vi "Master Setup Read Write Update Command.vi"(8 "error in (no error)":errorcluster, 9 "Read (F)/Write (T)":bool, 10 "Pattern Label":T1 items=["Channel Setup (0)", "PID Setup (1)", "Filter Setup (2)", "~Reserved Old CAN Msgs (3)", "~Reserved Old CAN1 (4)", "~Reserved Old CAN2 (5)", "Digital Inputs Setup (6)", "Digital Outputs Setup (7)", "Logging 1 Setup (8)", "Logging 2 Setup (9)", "Logging 3 Setup (10)", "Setpoint Setup (11)", "Test Series Setup (12)", "Graph Setup (13)", "System Configure (14)", "Header (15)", "Profile Manager (16)", "Post-Mortem Logging (17)", "High-Speed Data (18)", "Statistic Channel Setup (19)", "Ramp Channel Setup (20)", "ETAS INCA Channel Setup (21)", "ETC ECCS Transducer Setup (22)", "ETC ECCS Test Setup (23)", "AVL AK Smoke Meter Setup (24)", "Triggers Setup (25)", "Alarm Limits Setup (26)", "YKWT1 Measurement (27)", "YKWT1 Instrument (28)", "Auto File Settings (29)", "Playback File Setting (30)", "UUT Constants (31)", "UPS Setup (32)", "Differential Channel Setup (33)", "Integral Channel Setup (34)", "Signal Channel Setup (35)", "Calibration Setup (36)", "BNC Setup (37)", "ASAP3 Setup (38)", "Chassis Force Calculations (39)", "Chassis Teststand Losses (40)", "Chassis Vehicle Losses (41)", "Formula Channels (42)", "ASAP3 Map Coords Setup (43)", "Digital Controls Setup (44)", "Push Buttons Setup (45)", "Sliders Setup (46)", "~Reserved~ (47)", "Email Setup (48)", "Timer Setup (49)", "Unit Conversion Setup (50)", "Visible Channels (51)", "Main Display Setup (52)", "Message Display Setup (53)", "Input Display Setup (54)", "Unico Parameter Downloads (55)", "Flow Meter Setup (56)", "Channel Zero Offset (57)", "YKWT2 Measurement (58)", "YKWT2 Instrument (59)", "~Reserved Old CAN3 (60)", "CAS Setup (61)", "Accumulation Channel Setup (62)", "Valvetrain Dynamics Setup (63)", "CCP Setup (64)", "System Log Setup (65)", "Throttle Controller (66)", "RE Shifter (67)", "Main Display (68)", "~Reserved~ (69)", "FlexRay (70)", "YKWT3 Measurement (71)", "YKWT3 Instrument (72)", "CAN XNET API (73)"], 11 "Update Command (in)":bool) -> (0 "error out":errorcluster, 3 "Update Command (out)":bool)   [LabVIEW 2017]
uses:
  Master Setup Pattern Enum.ctl
panel:
  in  "Setup File (System Configure)":path=path "C:/Revolutionary Engineering/REPS/Setup Files/Default/GM Trans Cell 2/SystemConfigure GM cell 2.cfs"
  in  "Setup File (Setpoint)":path=path "C:/Revolutionary Engineering/REPS/Setup Files/Default/RE Cell 3-1/re cell 3 setpoints.spt"
  in  "Setup File (CAN 0)":path
  in  "Setup File (CAN 1)":path
  in  "Setup File (Can Message)":path
  in  "Setup File (Playback)":path
  in  "Setup File (UUT Constants)":path
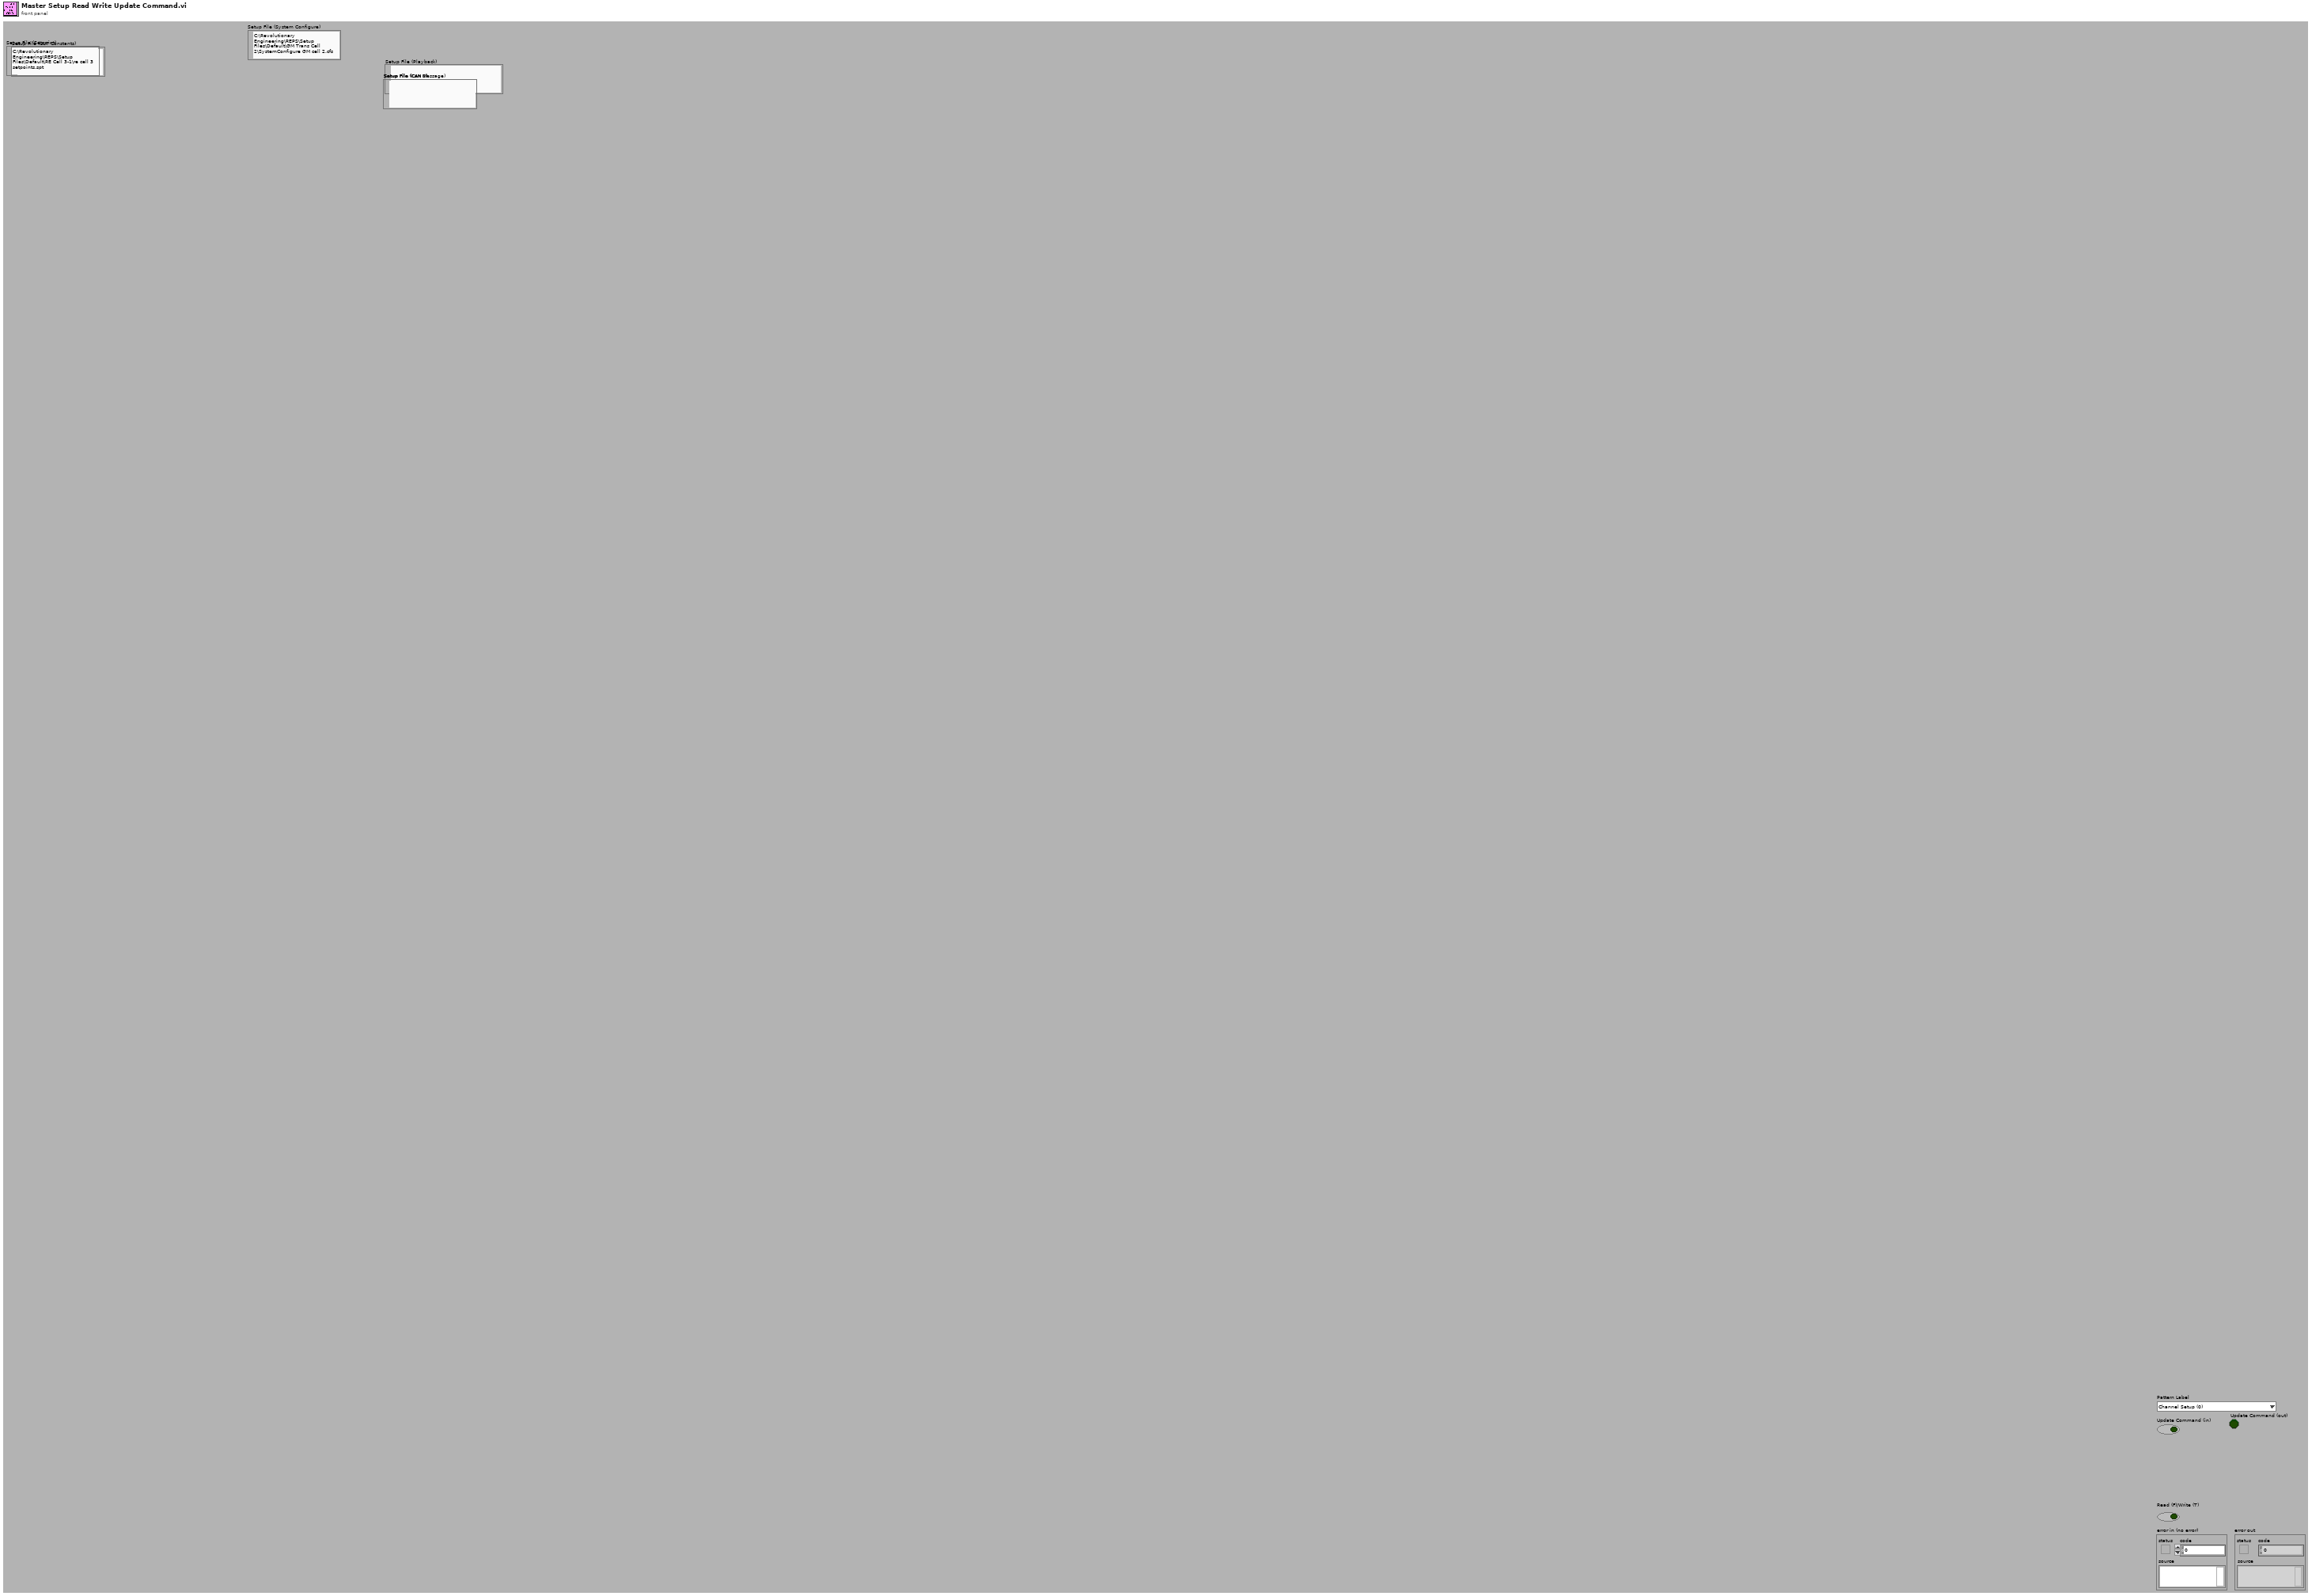
[diagram p1: front panel]
types:
  T1 = typedef "Master Setup Pattern Enum.ctl" = i32
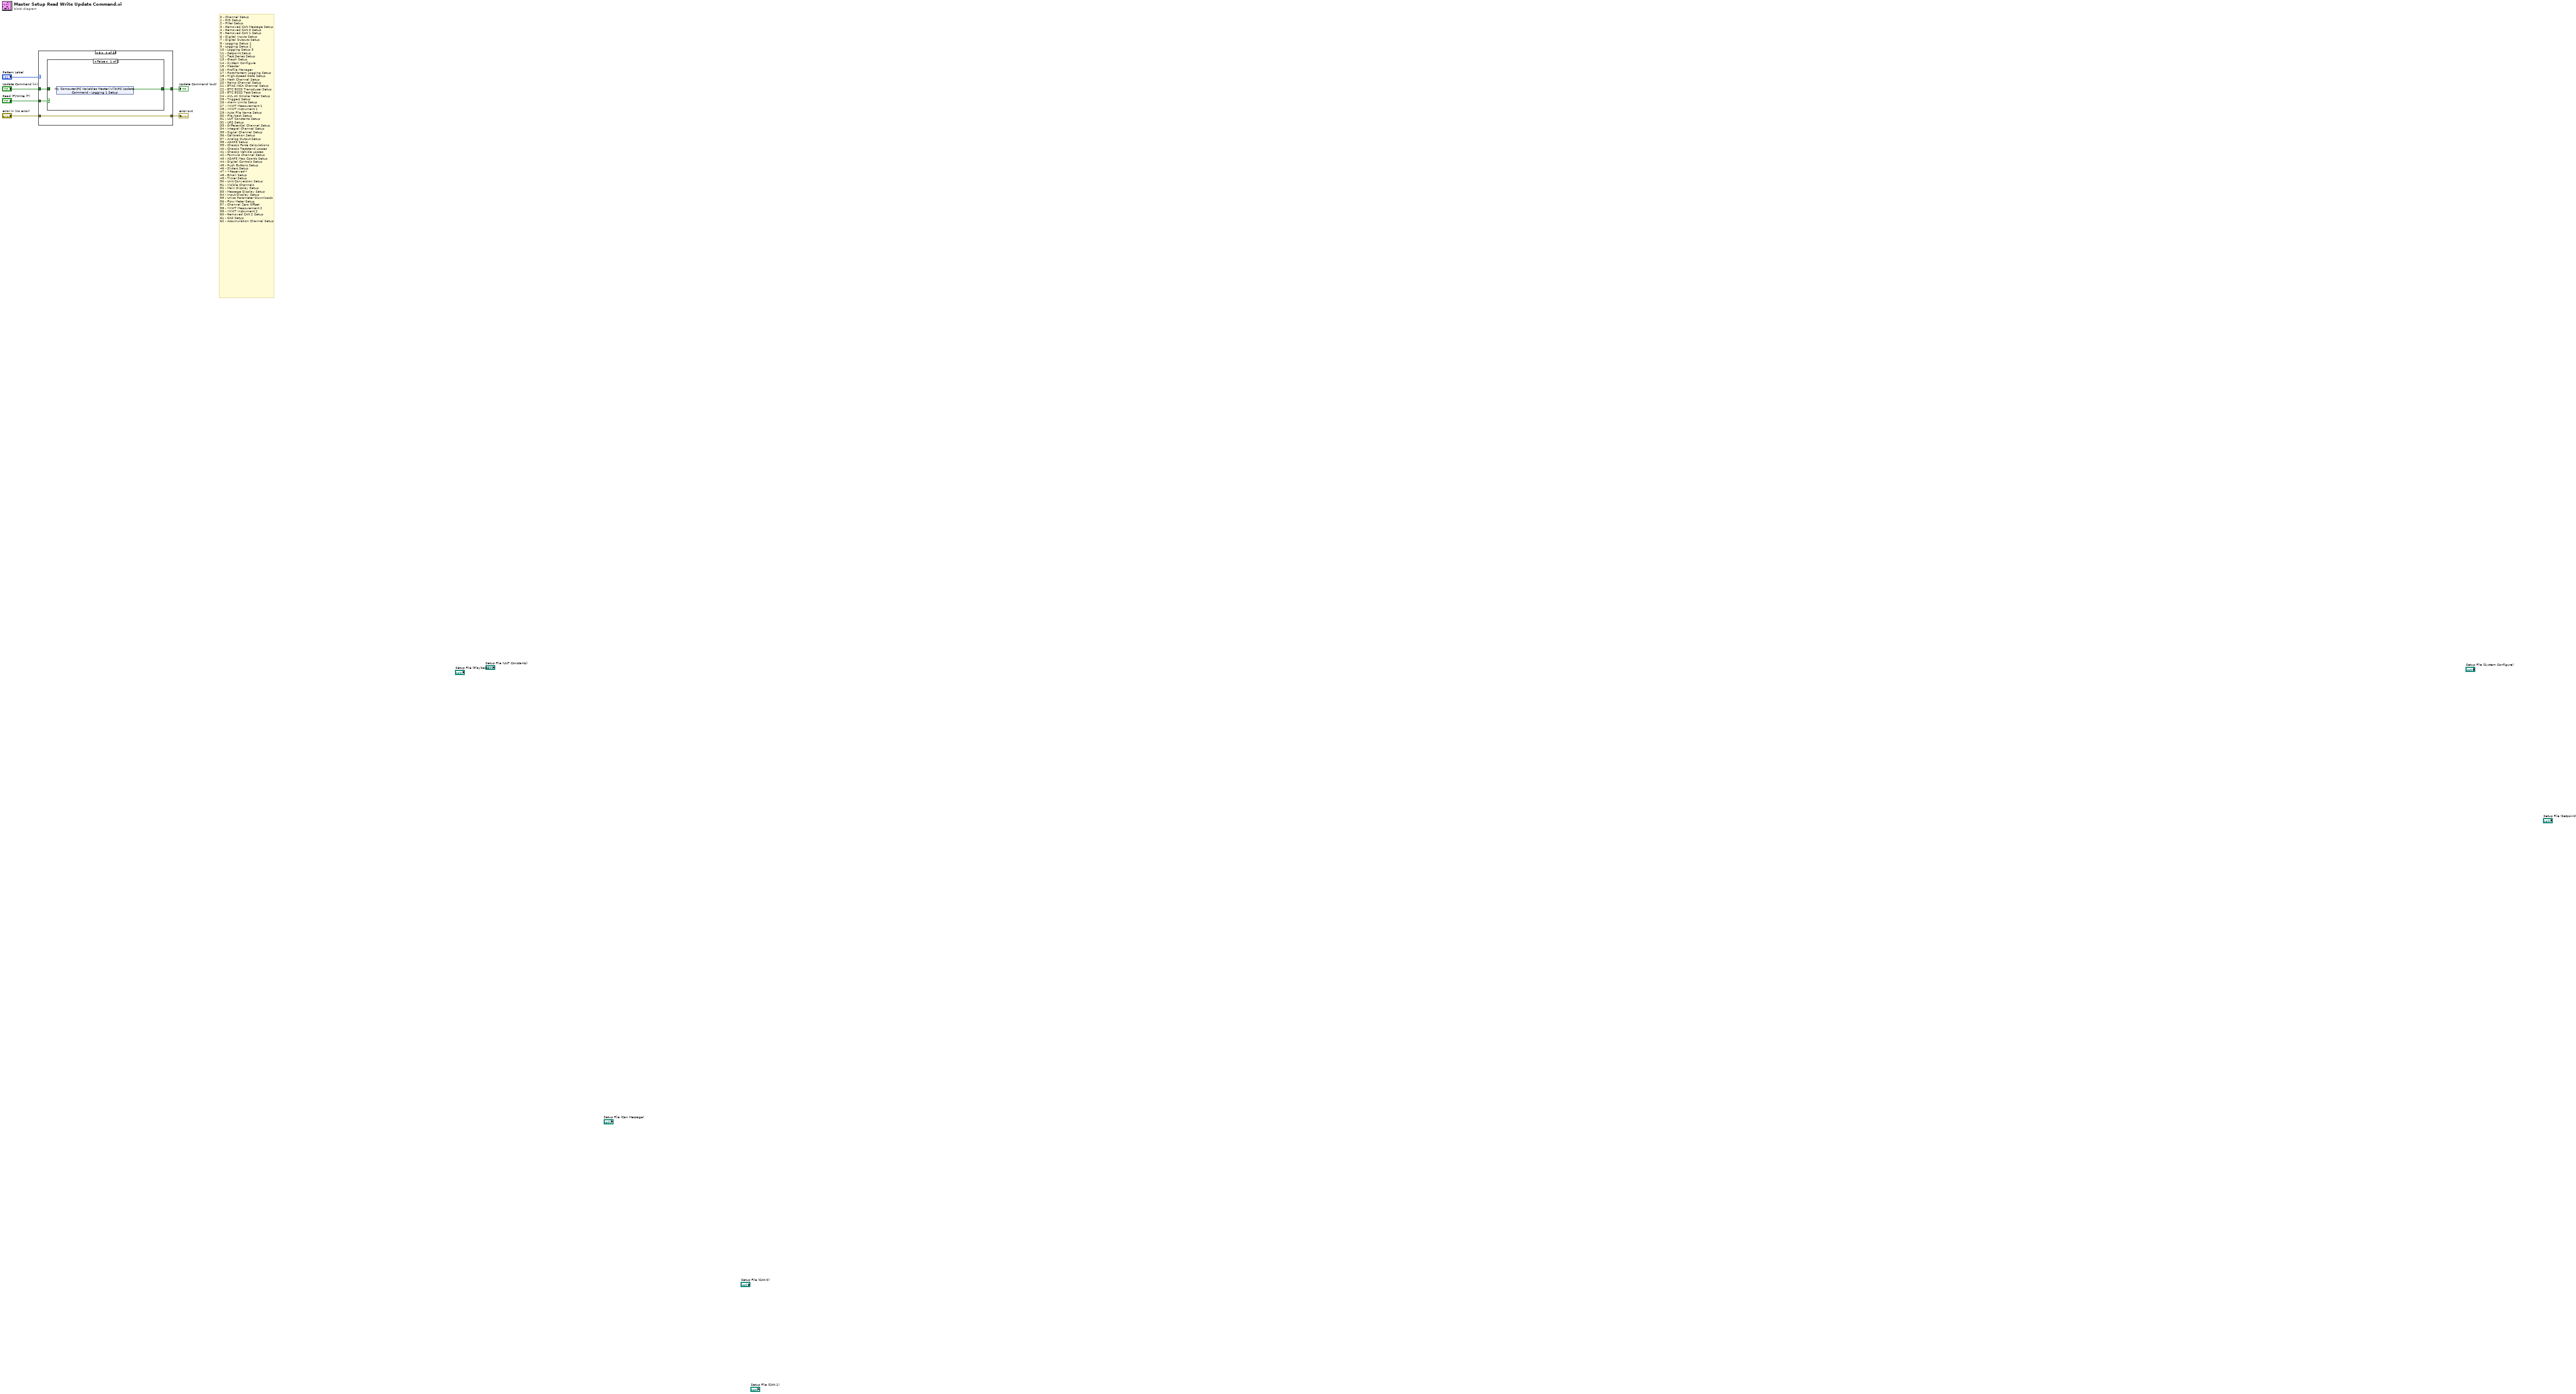
[diagram p0: block diagram]
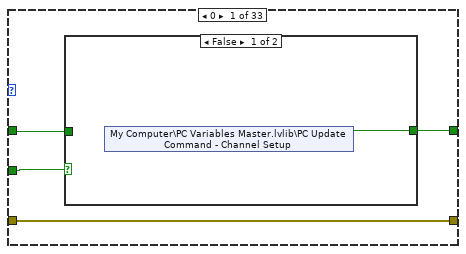
[diagram p2: hidden frame]
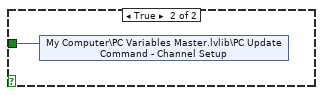
[diagram p3: hidden frame]
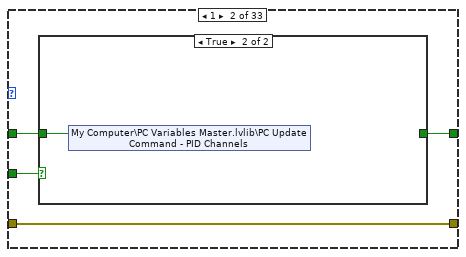
[diagram p4: hidden frame]
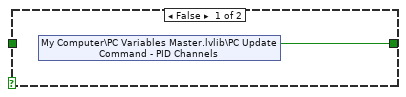
[diagram p5: hidden frame]
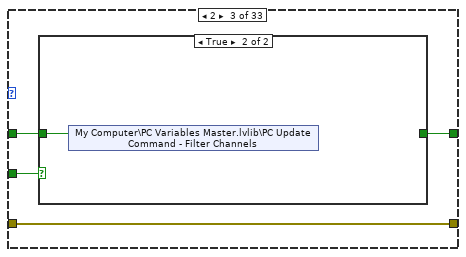
[diagram p6: hidden frame]
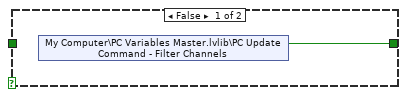
[diagram p7: hidden frame]
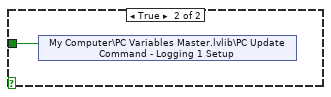
[diagram p8: hidden frame]
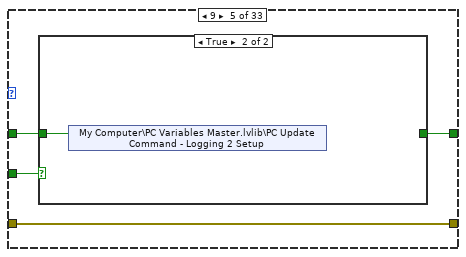
[diagram p9: hidden frame]
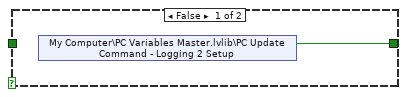
[diagram p10: hidden frame]
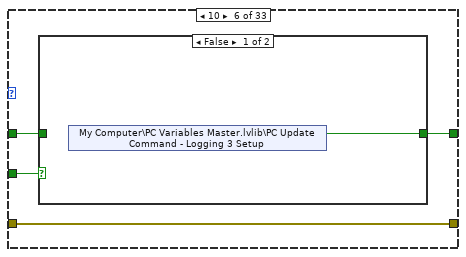
[diagram p11: hidden frame]
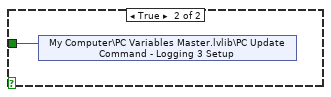
[diagram p12: hidden frame]
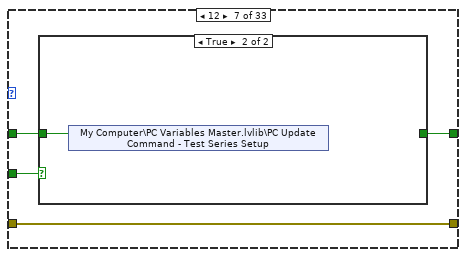
[diagram p13: hidden frame]
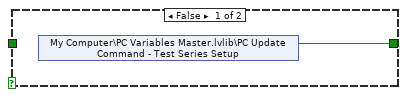
[diagram p14: hidden frame]
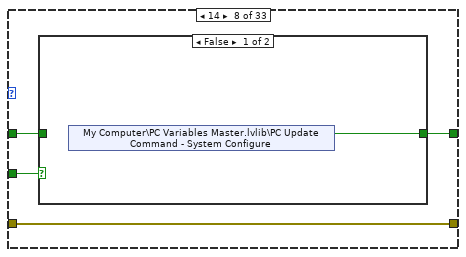
[diagram p15: hidden frame]
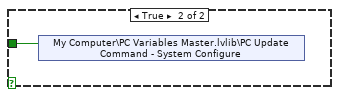
[diagram p16: hidden frame]
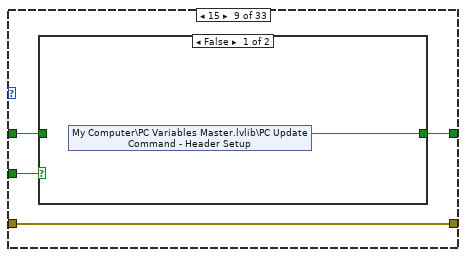
[diagram p17: hidden frame]
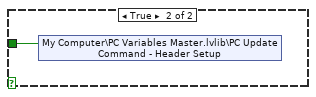
[diagram p18: hidden frame]
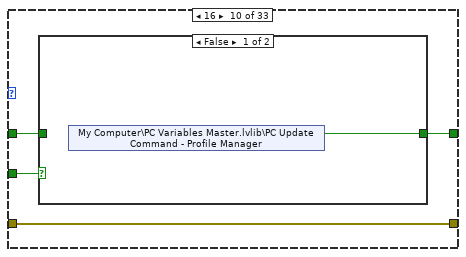
[diagram p19: hidden frame]
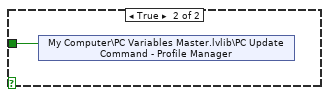
[diagram p20: hidden frame]
diagram:
  # "0 - Channel Setup\n1 - PID Setup\n2 - Filter Setup\n3 - Removed CAN Message Setup\n4 - Removed CAN 0 Setup\n5 - Removed CAN 1 Setup\n6 - Digital Inputs Setup\n7 - Digital Outputs Setup\n8 - Logging Setup 1\n9 - Logging Setup 2\n10 - Logging Setup 3\n11 - Setpoint Setup\n12 - Test Series Setup\n13 - Graph Setup\n14 - System Configure\n15 - Header\n16 - Profile Manager\n17 - Post-Mortem Logging Setup\n18 - High-Speed Data Setup\n19 - Math Channel Setup\n20 - Ramp Channel Setup\n21 - ETAS INCA Channel Setup\n22 - ETC ECCS Transducer Setup\n23 - ETC ECCS Test Setup\n24 - AVL AK Smoke Meter Setup\n25 - Triggers Setup\n26 - Alarm Limits Setup\n27 - YKWT Measurement 1\n28 - YKWT Instrument 1\n29 - Auto File Name Setup\n30 - Playback Setup\n31 - UUT Constants Setup\n32 - UPS Setup\n33 - Differential Channel Setup\n34 - Integral Channel Setup\n35 - Signal Channel Setup\n36 - Calibration Setup\n37 - Analog Output Setup\n38 - ASAP3 Setup\n39 - Chassis Force Calculations\n40 - Chassis Teststand Losses\n41 - Chassis Vehicle Losses\n42 - Formula Channel Setup\n43 - ASAP3 Map Coords Setup\n44 - Digital Controls Setup\n45 - Push Buttons Setup\n46 - Sliders Setup\n47 - ~Reserved~\n48 - Email Setup\n49 - Timer Setup\n50 - Unit Conversion Setup\n51 - Visible Channels\n52 - Main Display Setup\n53 - Message Display Setup\n54 - Input Display Setup\n55 - Unico Parameter Downloads\n56 - Flow Meter Setup\n57 - Channel Zero Offset\n58 - YKWT Measurement 2\n59 - YKWT Instrument 2\n60 - Removed CAN 2 Setup\n61 - CAS Setup\n62 - Accumulation Channel Setup"
  n1 = case shown="8" "Pattern Label" {
    tunnel: "Read (F)/Write (T)" -> [w10 w16 w22 w28 w34 w40 w46 w52 w58 w64 w70 w76 w82 w88 w94 w100 w106 w112 w118 w124 w130 w136 w142 w148 w154 w159 w166 w172 w178 w184 w190 w196 _]
    tunnel: "Update Command (in)" -> [w8 w15 w21 w27 w33 w39 w45 w51 w57 w63 w69 w75 w81 w87 w93 w99 w105 w111 w117 w123 w129 w135 w141 w147 w153 w158 w165 w170 w176 w182 w188 w194 _]
    tunnel: [w9 w14 w20 w26 w32 w38 w44 w50 w56 w62 w68 w74 w80 w86 w92 w98 w104 w110 w116 w122 w128 w134 w140 w146 w152 w157 w164 w171 w177 w183 w189 w195 _] -> w3
    tunnel: "error in (no error)" -> [w7 w13 w19 w25 w31 w37 w43 w49 w55 w61 w67 w73 w79 w85 w91 w97 w103 w109 w115 w121 w127 w133 w139 w145 w151 w160 w163 w169 w175 w181 w187 w193 w200]
    tunnel: [w7 w13 w19 w25 w31 w37 w43 w49 w55 w61 w67 w73 w79 w85 w91 w97 w103 w109 w115 w121 w127 w133 w139 w145 w151 w160 w163 w169 w175 w181 w187 w193 w199] -> w1
    frame 0 {
      n2 = case shown="False" w10 {
        tunnel: [w11 _] -> w9
        tunnel: w8 -> [_ w12]
        frame False {
          n3 = shared-variable "My Computer\\PC Variables Master.lvlib\\PC Update Command - Channel Setup"() -> (w11:bool)  [unwired: 1 in, 1 out]
        }
        frame True {
          n4 = shared-variable "My Computer\\PC Variables Master.lvlib\\PC Update Command - Channel Setup"(w12) -> ()  [unwired: 1 in, 1 out]
        }
      }
    }
    frame 1 {
      n5 = case shown="True" w16 {
        tunnel: w15 -> [_ w18]
        tunnel: [w17 _] -> w14
        frame False {
          n6 = shared-variable "My Computer\\PC Variables Master.lvlib\\PC Update Command - PID Channels"() -> (w17:bool)  [unwired: 1 in, 1 out]
        }
        frame True {
          n7 = shared-variable "My Computer\\PC Variables Master.lvlib\\PC Update Command - PID Channels"(w18) -> ()  [unwired: 1 in, 1 out]
        }
      }
    }
    frame 2 {
      n8 = case shown="True" w22 {
        tunnel: w21 -> [_ w24]
        tunnel: [w23 _] -> w20
        frame False {
          n9 = shared-variable "My Computer\\PC Variables Master.lvlib\\PC Update Command - Filter Channels"() -> (w23:bool)  [unwired: 1 in, 1 out]
        }
        frame True {
          n10 = shared-variable "My Computer\\PC Variables Master.lvlib\\PC Update Command - Filter Channels"(w24) -> ()  [unwired: 1 in, 1 out]
        }
      }
    }
    frame 8 {
      n11 = case shown="False" w28 {
        tunnel: w27 -> [_ w30]
        tunnel: [w29 _] -> w26
        frame False {
          n12 = shared-variable "My Computer\\PC Variables Master.lvlib\\PC Update Command - Logging 1 Setup"() -> (w29:bool)  [unwired: 1 in, 1 out]
        }
        frame True {
          n13 = shared-variable "My Computer\\PC Variables Master.lvlib\\PC Update Command - Logging 1 Setup"(w30) -> ()  [unwired: 1 in, 1 out]
        }
      }
    }
    frame 9 {
      n14 = case shown="True" w34 {
        tunnel: w33 -> [_ w36]
        tunnel: [w35 _] -> w32
        frame False {
          n15 = shared-variable "My Computer\\PC Variables Master.lvlib\\PC Update Command - Logging 2 Setup"() -> (w35:bool)  [unwired: 1 in, 1 out]
        }
        frame True {
          n16 = shared-variable "My Computer\\PC Variables Master.lvlib\\PC Update Command - Logging 2 Setup"(w36) -> ()  [unwired: 1 in, 1 out]
        }
      }
    }
    frame 10 {
      n17 = case shown="False" w40 {
        tunnel: w39 -> [_ w42]
        tunnel: [w41 _] -> w38
        frame False {
          n18 = shared-variable "My Computer\\PC Variables Master.lvlib\\PC Update Command - Logging 3 Setup"() -> (w41:bool)  [unwired: 1 in, 1 out]
        }
        frame True {
          n19 = shared-variable "My Computer\\PC Variables Master.lvlib\\PC Update Command - Logging 3 Setup"(w42) -> ()  [unwired: 1 in, 1 out]
        }
      }
    }
    frame 12 {
      n20 = case shown="True" w46 {
        tunnel: w45 -> [_ w48]
        tunnel: [w47 _] -> w44
        frame False {
          n21 = shared-variable "My Computer\\PC Variables Master.lvlib\\PC Update Command - Test Series Setup"() -> (w47:bool)  [unwired: 1 in, 1 out]
        }
        frame True {
          n22 = shared-variable "My Computer\\PC Variables Master.lvlib\\PC Update Command - Test Series Setup"(w48) -> ()  [unwired: 1 in, 1 out]
        }
      }
    }
    frame 14 {
      n23 = case shown="False" w52 {
        tunnel: w51 -> [_ w54]
        tunnel: [w53 _] -> w50
        frame False {
          n24 = shared-variable "My Computer\\PC Variables Master.lvlib\\PC Update Command - System Configure"() -> (w53:bool)  [unwired: 1 in, 1 out]
        }
        frame True {
          n25 = shared-variable "My Computer\\PC Variables Master.lvlib\\PC Update Command - System Configure"(w54) -> ()  [unwired: 1 in, 1 out]
        }
      }
    }
    frame 15 {
      n26 = case shown="False" w58 {
        tunnel: w57 -> [_ w60]
        tunnel: [w59 _] -> w56
        frame False {
          n27 = shared-variable "My Computer\\PC Variables Master.lvlib\\PC Update Command - Header Setup"() -> (w59:bool)  [unwired: 1 in, 1 out]
        }
        frame True {
          n28 = shared-variable "My Computer\\PC Variables Master.lvlib\\PC Update Command - Header Setup"(w60) -> ()  [unwired: 1 in, 1 out]
        }
      }
    }
    frame 16 {
      n29 = case shown="False" w64 {
        tunnel: w63 -> [_ w66]
        tunnel: [w65 _] -> w62
        frame False {
          n30 = shared-variable "My Computer\\PC Variables Master.lvlib\\PC Update Command - Profile Manager"() -> (w65:bool)  [unwired: 1 in, 1 out]
        }
        frame True {
          n31 = shared-variable "My Computer\\PC Variables Master.lvlib\\PC Update Command - Profile Manager"(w66) -> ()  [unwired: 1 in, 1 out]
        }
      }
    }
    frame 17 {
      n32 = case shown="True" w70 {
        tunnel: w69 -> [_ w72]
        tunnel: [w71 _] -> w68
        frame False {
          n33 = shared-variable "My Computer\\PC Variables Master.lvlib\\PC Update Command - Logging PM Setup"() -> (w71:bool)  [unwired: 1 in, 1 out]
        }
        frame True {
          n34 = shared-variable "My Computer\\PC Variables Master.lvlib\\PC Update Command - Logging PM Setup"(w72) -> ()  [unwired: 1 in, 1 out]
        }
      }
    }
    frame 19 {
      n35 = case shown="True" w76 {
        tunnel: w75 -> [_ w78]
        tunnel: [w77 _] -> w74
        frame False {
          n36 = shared-variable "My Computer\\PC Variables Master.lvlib\\PC Update Command - Math Channels"() -> (w77:bool)  [unwired: 1 in, 1 out]
        }
        frame True {
          n37 = shared-variable "My Computer\\PC Variables Master.lvlib\\PC Update Command - Math Channels"(w78) -> ()  [unwired: 1 in, 1 out]
        }
      }
    }
    frame 20 {
      n38 = case shown="False" w82 {
        tunnel: w81 -> [_ w84]
        tunnel: [w83 _] -> w80
        frame False {
          n39 = shared-variable "My Computer\\PC Variables Master.lvlib\\PC Update Command - Ramp Channels"() -> (w83:bool)  [unwired: 1 in, 1 out]
        }
        frame True {
          n40 = shared-variable "My Computer\\PC Variables Master.lvlib\\PC Update Command - Ramp Channels"(w84) -> ()  [unwired: 1 in, 1 out]
        }
      }
    }
    frame 25 {
      n41 = case shown="True" w88 {
        tunnel: w87 -> [_ w90]
        tunnel: [w89 _] -> w86
        frame False {
          n42 = shared-variable "My Computer\\PC Variables Master.lvlib\\PC Update Command - Trigger Channels"() -> (w89:bool)  [unwired: 1 in, 1 out]
        }
        frame True {
          n43 = shared-variable "My Computer\\PC Variables Master.lvlib\\PC Update Command - Trigger Channels"(w90) -> ()  [unwired: 1 in, 1 out]
        }
      }
    }
    frame 26 {
      n44 = case shown="False" w94 {
        tunnel: w93 -> [_ w96]
        tunnel: [w95 _] -> w92
        frame False {
          n45 = shared-variable "My Computer\\PC Variables Master.lvlib\\PC Update Command - Alarm Limits Setup"() -> (w95:bool)  [unwired: 1 in, 1 out]
        }
        frame True {
          n46 = shared-variable "My Computer\\PC Variables Master.lvlib\\PC Update Command - Alarm Limits Setup"(w96) -> ()  [unwired: 1 in, 1 out]
        }
      }
    }
    frame 30 {
      n47 = case shown="True" w100 {
        tunnel: w99 -> [_ w102]
        tunnel: [w101 _] -> w98
        frame False {
          n48 = shared-variable "My Computer\\PC Variables Master.lvlib\\PC Update Command - Playback Setup"() -> (w101:bool)  [unwired: 1 in, 1 out]
        }
        frame True {
          n49 = shared-variable "My Computer\\PC Variables Master.lvlib\\PC Update Command - Playback Setup"(w102) -> ()  [unwired: 1 in, 1 out]
        }
      }
    }
    frame 33 {
      n50 = case shown="True" w106 {
        tunnel: w105 -> [_ w108]
        tunnel: [w107 _] -> w104
        frame False {
          n51 = shared-variable "My Computer\\PC Variables Master.lvlib\\PC Update Command - Differential Channels"() -> (w107:bool)  [unwired: 1 in, 1 out]
        }
        frame True {
          n52 = shared-variable "My Computer\\PC Variables Master.lvlib\\PC Update Command - Differential Channels"(w108) -> ()  [unwired: 1 in, 1 out]
        }
      }
    }
    frame 34 {
      n53 = case shown="False" w112 {
        tunnel: w111 -> [_ w114]
        tunnel: [w113 _] -> w110
        frame False {
          n54 = shared-variable "My Computer\\PC Variables Master.lvlib\\PC Update Command - Integration Channels"() -> (w113:bool)  [unwired: 1 in, 1 out]
        }
        frame True {
          n55 = shared-variable "My Computer\\PC Variables Master.lvlib\\PC Update Command - Integration Channels"(w114) -> ()  [unwired: 1 in, 1 out]
        }
      }
    }
    frame 35 {
      n56 = case shown="True" w118 {
        tunnel: w117 -> [_ w120]
        tunnel: [w119 _] -> w116
        frame False {
          n57 = shared-variable "My Computer\\PC Variables Master.lvlib\\PC Update Command - Waveform Signal Channels"() -> (w119:bool)  [unwired: 1 in, 1 out]
        }
        frame True {
          n58 = shared-variable "My Computer\\PC Variables Master.lvlib\\PC Update Command - Waveform Signal Channels"(w120) -> ()  [unwired: 1 in, 1 out]
        }
      }
    }
    frame 36 {
      n59 = case shown="False" w124 {
        tunnel: w123 -> [_ w126]
        tunnel: [w125 _] -> w122
        frame False {
          n60 = shared-variable "My Computer\\PC Variables Master.lvlib\\PC Update Command - Calibration Setup"() -> (w125:bool)  [unwired: 1 in, 1 out]
        }
        frame True {
          n61 = shared-variable "My Computer\\PC Variables Master.lvlib\\PC Update Command - Calibration Setup"(w126) -> ()  [unwired: 1 in, 1 out]
        }
      }
    }
    frame 37 {
      n62 = case shown="True" w130 {
        tunnel: w129 -> [_ w132]
        tunnel: [w131 _] -> w128
        frame False {
          n63 = shared-variable "My Computer\\PC Variables Master.lvlib\\PC Update Command - BNC Setup"() -> (w131:bool)  [unwired: 1 in, 1 out]
        }
        frame True {
          n64 = shared-variable "My Computer\\PC Variables Master.lvlib\\PC Update Command - BNC Setup"(w132) -> ()  [unwired: 1 in, 1 out]
        }
      }
    }
    frame 42 {
      n65 = case shown="True" w136 {
        tunnel: w135 -> [_ w138]
        tunnel: [w137 _] -> w134
        frame False {
          n66 = shared-variable "My Computer\\PC Variables Master.lvlib\\PC Update Command - Formula Channels"() -> (w137:bool)  [unwired: 1 in, 1 out]
        }
        frame True {
          n67 = shared-variable "My Computer\\PC Variables Master.lvlib\\PC Update Command - Formula Channels"(w138) -> ()  [unwired: 1 in, 1 out]
        }
      }
    }
    frame 45 {
      n68 = case shown="True" w142 {
        tunnel: w141 -> [_ w144]
        tunnel: [w143 _] -> w140
        frame False {
          n69 = shared-variable "My Computer\\PC Variables Master.lvlib\\PC Update Command - Push Button Setup"() -> (w143:bool)  [unwired: 1 in, 1 out]
        }
        frame True {
          n70 = shared-variable "My Computer\\PC Variables Master.lvlib\\PC Update Command - Push Button Setup"(w144) -> ()  [unwired: 1 in, 1 out]
        }
      }
    }
    frame 49 {
      n71 = case shown="True" w148 {
        tunnel: w147 -> [_ w150]
        tunnel: [w149 _] -> w146
        frame False {
          n72 = shared-variable "My Computer\\PC Variables Master.lvlib\\PC Update Command - Timer Channels"() -> (w149:bool)  [unwired: 1 in, 1 out]
        }
        frame True {
          n73 = shared-variable "My Computer\\PC Variables Master.lvlib\\PC Update Command - Timer Channels"(w150) -> ()  [unwired: 1 in, 1 out]
        }
      }
    }
    frame 50 {
      n74 = case shown="True" w154 {
        tunnel: w153 -> [_ w156]
        tunnel: [w155 _] -> w152
        frame False {
          n75 = shared-variable "My Computer\\PC Variables Master.lvlib\\PC Update Command - Unit Conversion"() -> (w155:bool)  [unwired: 1 in, 1 out]
        }
        frame True {
          n76 = shared-variable "My Computer\\PC Variables Master.lvlib\\PC Update Command - Unit Conversion"(w156) -> ()  [unwired: 1 in, 1 out]
        }
      }
    }
    frame 56 {
      n77 = case shown="False" w159 {
        tunnel: w158 -> [_ w162]
        tunnel: [w161 _] -> w157
        frame False {
          n78 = shared-variable "My Computer\\PC Variables Master.lvlib\\PC Update Command - Flow Meter Channels"() -> (w161:bool)  [unwired: 1 in, 1 out]
        }
        frame True {
          n79 = shared-variable "My Computer\\PC Variables Master.lvlib\\PC Update Command - Flow Meter Channels"(w162) -> ()  [unwired: 1 in, 1 out]
        }
      }
    }
    frame 57 {
      n80 = case shown="False" w166 {
        tunnel: w165 -> [_ w168]
        tunnel: [w167 _] -> w164
        frame False {
          n81 = shared-variable "My Computer\\PC Variables Master.lvlib\\PC Update Command - Zero Offset Setup"() -> (w167:bool)  [unwired: 1 in, 1 out]
        }
        frame True {
          n82 = shared-variable "My Computer\\PC Variables Master.lvlib\\PC Update Command - Zero Offset Setup"(w168) -> ()  [unwired: 1 in, 1 out]
        }
      }
    }
    frame 62 {
      n83 = case shown="True" w172 {
        tunnel: [w173 _] -> w171
        tunnel: w170 -> [_ w174]
        frame False {
          n84 = shared-variable "My Computer\\PC Variables Master.lvlib\\PC Update Command - Accumulation Channels"() -> (w173:bool)  [unwired: 1 in, 1 out]
        }
        frame True {
          n85 = shared-variable "My Computer\\PC Variables Master.lvlib\\PC Update Command - Accumulation Channels"(w174) -> ()  [unwired: 1 in, 1 out]
        }
      }
    }
    frame 65 {
      n86 = case shown="False" w178 {
        tunnel: [w179 _] -> w177
        tunnel: w176 -> [_ w180]
        frame False {
          n87 = shared-variable "My Computer\\PC Variables Master.lvlib\\PC Update Command - System Log"() -> (w179:bool)  [unwired: 1 in, 1 out]
        }
        frame True {
          n88 = shared-variable "My Computer\\PC Variables Master.lvlib\\PC Update Command - System Log"(w180) -> ()  [unwired: 1 in, 1 out]
        }
      }
    }
    frame 64 {
      n89 = case shown="True" w184 {
        tunnel: [w185 _] -> w183
        tunnel: w182 -> [_ w186]
        frame False {
          n90 = shared-variable "My Computer\\PC Variables Master.lvlib\\PC Update Command - CCP"() -> (w185:bool)  [unwired: 1 in, 1 out]
        }
        frame True {
          n91 = shared-variable "My Computer\\PC Variables Master.lvlib\\PC Update Command - CCP"(w186) -> ()  [unwired: 1 in, 1 out]
        }
      }
    }
    frame 70 {
      n92 = case shown="False" w190 {
        tunnel: [w191 _] -> w189
        tunnel: w188 -> [_ w192]
        frame False {
          n93 = shared-variable "My Computer\\PC Variables Master.lvlib\\PC Update Command - FlexRay"() -> (w191:bool)  [unwired: 1 in, 1 out]
        }
        frame True {
          n94 = shared-variable "My Computer\\PC Variables Master.lvlib\\PC Update Command - FlexRay"(w192) -> ()  [unwired: 1 in, 1 out]
        }
      }
    }
    frame 73 {
      n95 = case shown="True" w196 {
        tunnel: [w197 _] -> w195
        tunnel: w194 -> [_ w198]
        frame False {
          n96 = shared-variable "My Computer\\PC Variables Master.lvlib\\PC Update Command - CAN XNET API"() -> (w197:bool)  [unwired: 1 in, 1 out]
        }
        frame True {
          n97 = shared-variable "My Computer\\PC Variables Master.lvlib\\PC Update Command - CAN XNET API"(w198) -> ()  [unwired: 1 in, 1 out]
        }
      }
    }
    frame Default {
      n98 = Select(t=w200, s=w200, f=errorcluster {"status"=TRUE, "code"=0, "source"=""}) -> (s? t:f=w199:errorcluster)
    }
  }
  "Update Command (out)" <- w3
  "error out" <- w1
